vi "close v2.vi"(8 "error in (no error)":errorcluster, 11 "para0":u64) -> (0 "error out":errorcluster)   [LabVIEW 2020, in "sqlite3.lvlib"]
uses:
  sqlite3.lvlib
  errstr.vi
  bin/sqlite3_64.dll
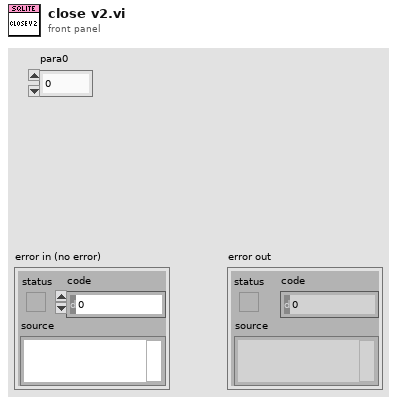
[diagram p1: front panel]
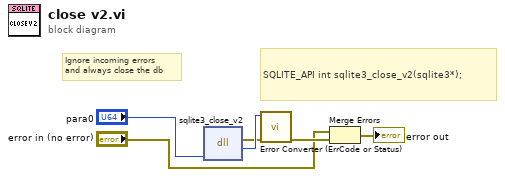
[diagram p0: block diagram]
diagram:
  # "Ignore incoming errors\nand always close the db"
  # "SQLITE_API int sqlite3_close_v2(sqlite3*);"
  n1 = dll-call lib="D:/Project/Labview-Projects/database-configuration/externals/sqlite3/Source/bin/sqlite3_*.*" fn="sqlite3_close_v2"("para0"="para0") -> (error out=w4:errorcluster, "return type"=w6:i32)  [unwired: 4 in, 1 out]
  n2 = call "Error Converter (ErrCode or Status).vi"("error in (no error)"=w4, "error code"=w6) -> ("error out"=w3:errorcluster)  [unwired: 9 in]
  n3 = Merge Errors("error in (no error)", w3) -> (→"error out":errorcluster)
